vi "Force Gate Update On XY Chart.vi"(8 "error in (no error)":errorcluster, 10 "Set?":bool caption="Set? (def: F - Read)", 11 "Test No.":u32) -> (0 "error out":errorcluster, 2 "Update gate display?":bool, 3 "Test No. out":u32)   [LabVIEW 2026, in "MicroPulse_Driver.lvlib"]
uses:
  MicroPulse_Driver.lvlib
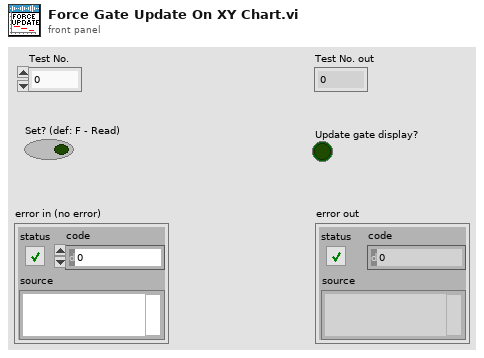
[diagram p1: front panel]
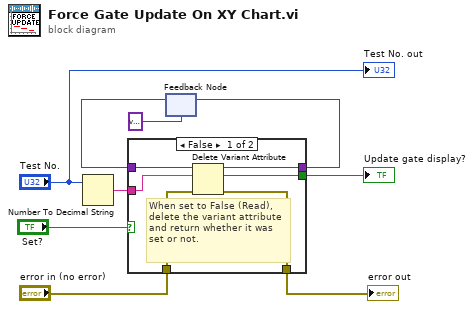
[diagram p0: block diagram]
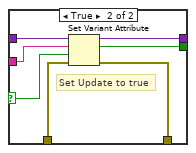
[diagram p2: hidden frame]
diagram:
  n1 = Number To Decimal String(number="Test No.") -> (decimal integer string=w7:string)  [unwired: 1 in]
  n2 = feedback #1(variant) -> (w6:variant)
  n3 = case shown="False" "Set?" {
    selector: "Set?" -> [_ w20]
    tunnel: w6 -> [w15 w22]
    tunnel: w7 -> [w13 w21]
    tunnel: [w14 w19] -> w8
    tunnel: [w12 w18] -> w9
    tunnel: "error in (no error)" -> [w11 w17]
    tunnel: [w10 w16] -> w1
    frame False {
      # "When set to False (Read), delete the variant attribute\nand return whether it was\nset or not."
      n4 = Delete Variant Attribute(4:w11, 6:w13, 7:w15) -> (0:w10:errorcluster, 2:w12:bool, 3:w14:variant)
    }
    frame True {
      # "Set Update to true"
      n5 = Set Variant Attribute(Variant=w22, name=w21, value=w20, error in=w17) -> (Variant out=w19:variant, replaced=w18:bool, error out=w16:errorcluster)
    }
  }
  "Update gate display?" <- w9
  "error out" <- w1
  n6 = feedback-in #1(w8) -> ()
  "Test No. out" <- "Test No."
